vi "Torque_and_Power_and_Doppler.vi"() -> ()   [LabVIEW 2020]
doc: "I. Description:\nThis example demonstrates how to continuously acquire data (Waveform) using the DAQ device's internal clock and an analog slope start trigger.\n\nII. Instructions for Running:\n1. Select the physical channel to correspond to where your signal is input on the DAQ device.\n2. Enter the minimum and maximum voltage ranges.\nNote: For better accuracy try to match the Input Ranges to the expected voltage level of the measured signal.\n3. Set the rate of the acquisition. Also set the Samples to Read control. This will determine how many samples are read each time the while loop iterates. This also determines how many points are plotted on the graph each iteration.\nNote: The rate should be at least twice as fast as the maximum frequency component of the signal being acquired.\n4. Set the source of the Analog Slope Start Trigger.\n5. Set the slope and level of desired analog edge condition.\n\nIII. Block Diagram Steps:\n1. Create an analog input voltage channel.\n2. Set the rate for the sample clock. Additionally, define the sample mode to be continuous.\n3. Define the parameters for an Analog Slope Start Trigger.\n4. Call the Start VI to start the acquisition.\n5. Read the waveform data in a loop until the user hits the stop button or an error occurs.\n6. Call the Clear Task VI to clear the Task.\n7. Use the popup dialog box to display an error if any.\n\nIV. I/O Connections Overview:\nMake sure your signal input terminal matches the Physical Channel I/O control. Also, make sure your analog trigger terminal matches the Trigger Source Control. For further connection information, refer to your hardware reference manual."
uses:
  <extravilib>/ChannelInstances/Tag-bool/Read With Abort.vi
  <extravilib>/ChannelInstances/Tag-bool/Write With Abort.vi
  <extravilib>/ChannelInstances/Tag-bool/Instantiate.vi
  <extravilib>/ChannelInstances/Tag-bool/EndpointRead.vi
  <extravilib>/ChannelInstances/Tag-bool/Endpoint.vi
  <extravilib>/ChannelInstances/Tag-bool.lvlib
panel:
  in  "stop 3":bool
  out "Feet Count":u64
  out "Pulses":u64
  out "Voltage":dynamicdata(graph)
  out "Current":dynamicdata(graph)
  out "Torque":dynamicdata(graph)
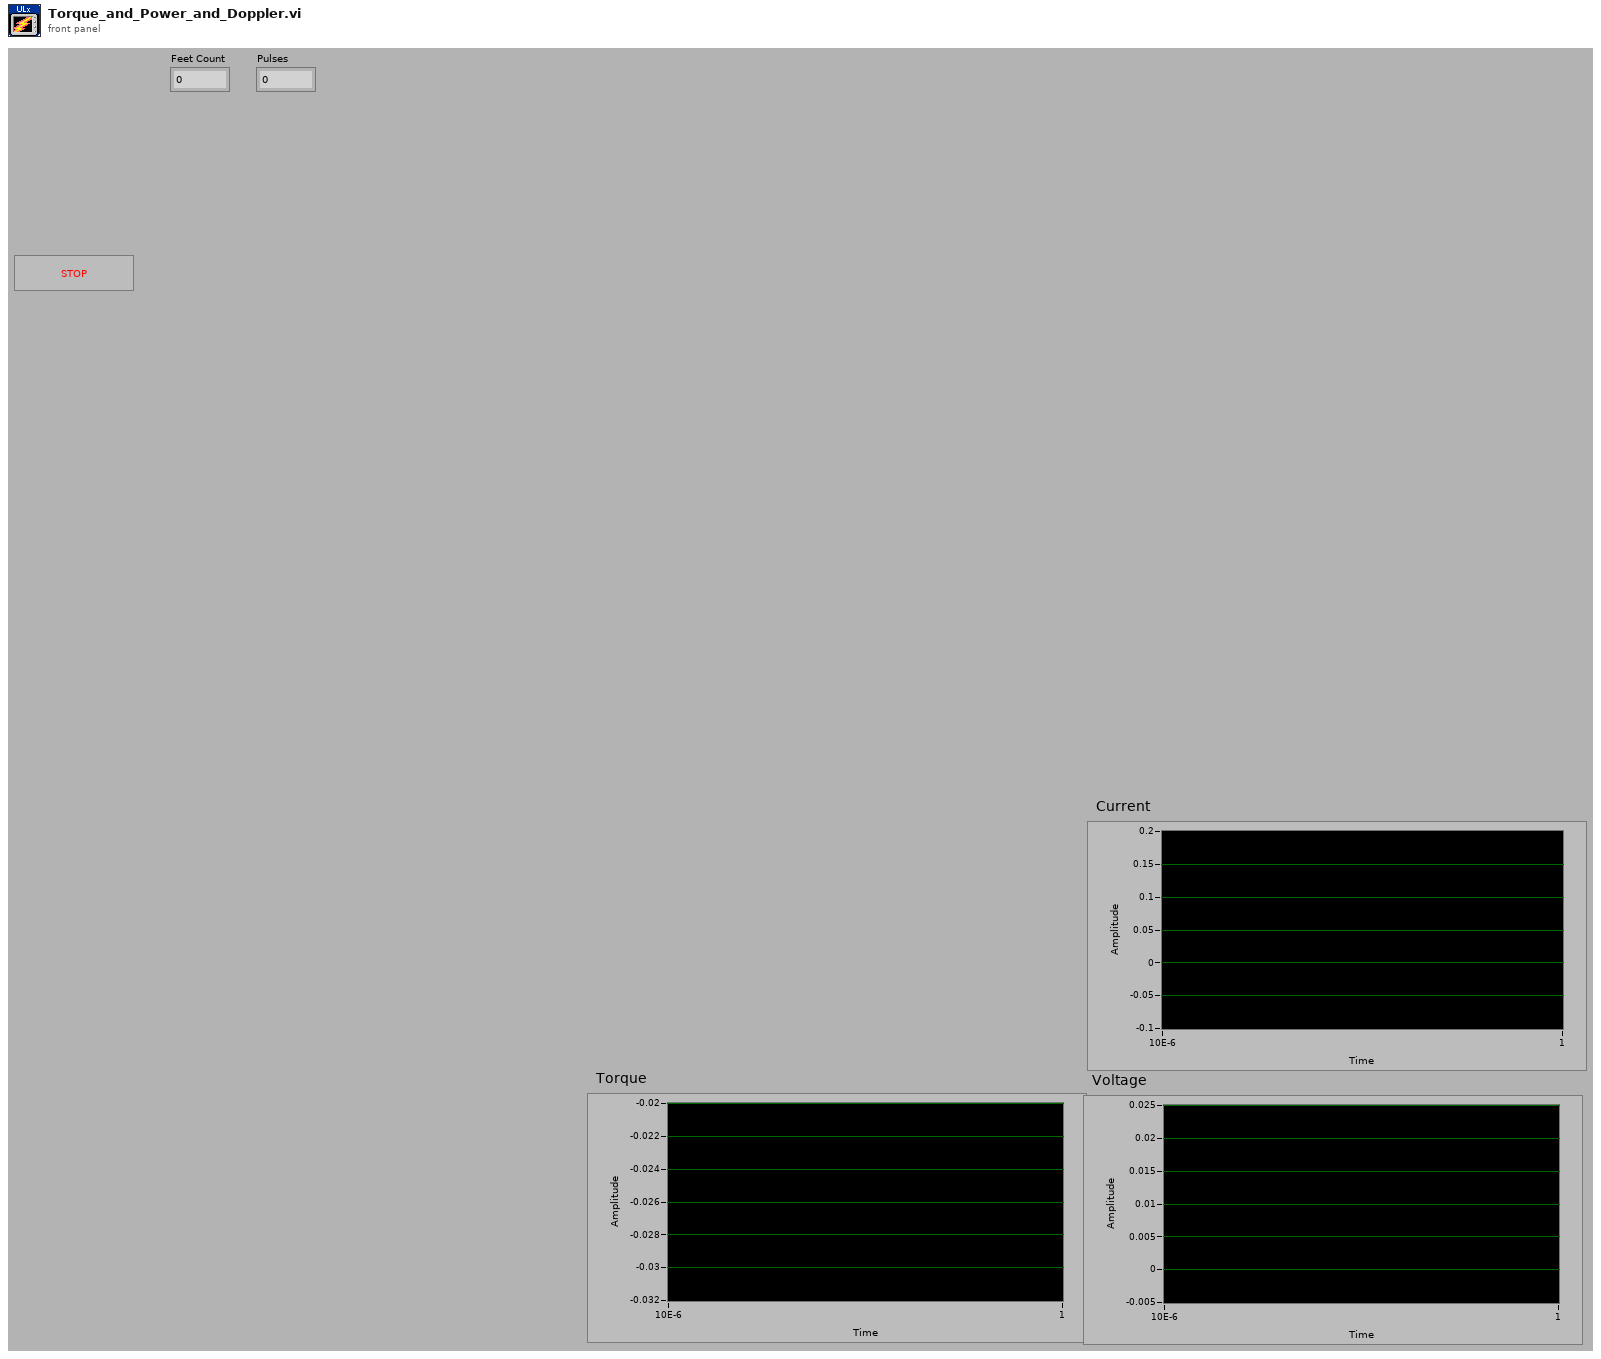
[diagram p1: front panel]
types:
  T1 = typedef "Tag-bool.lvlib/))Channel.ctl" = refnum<queue>
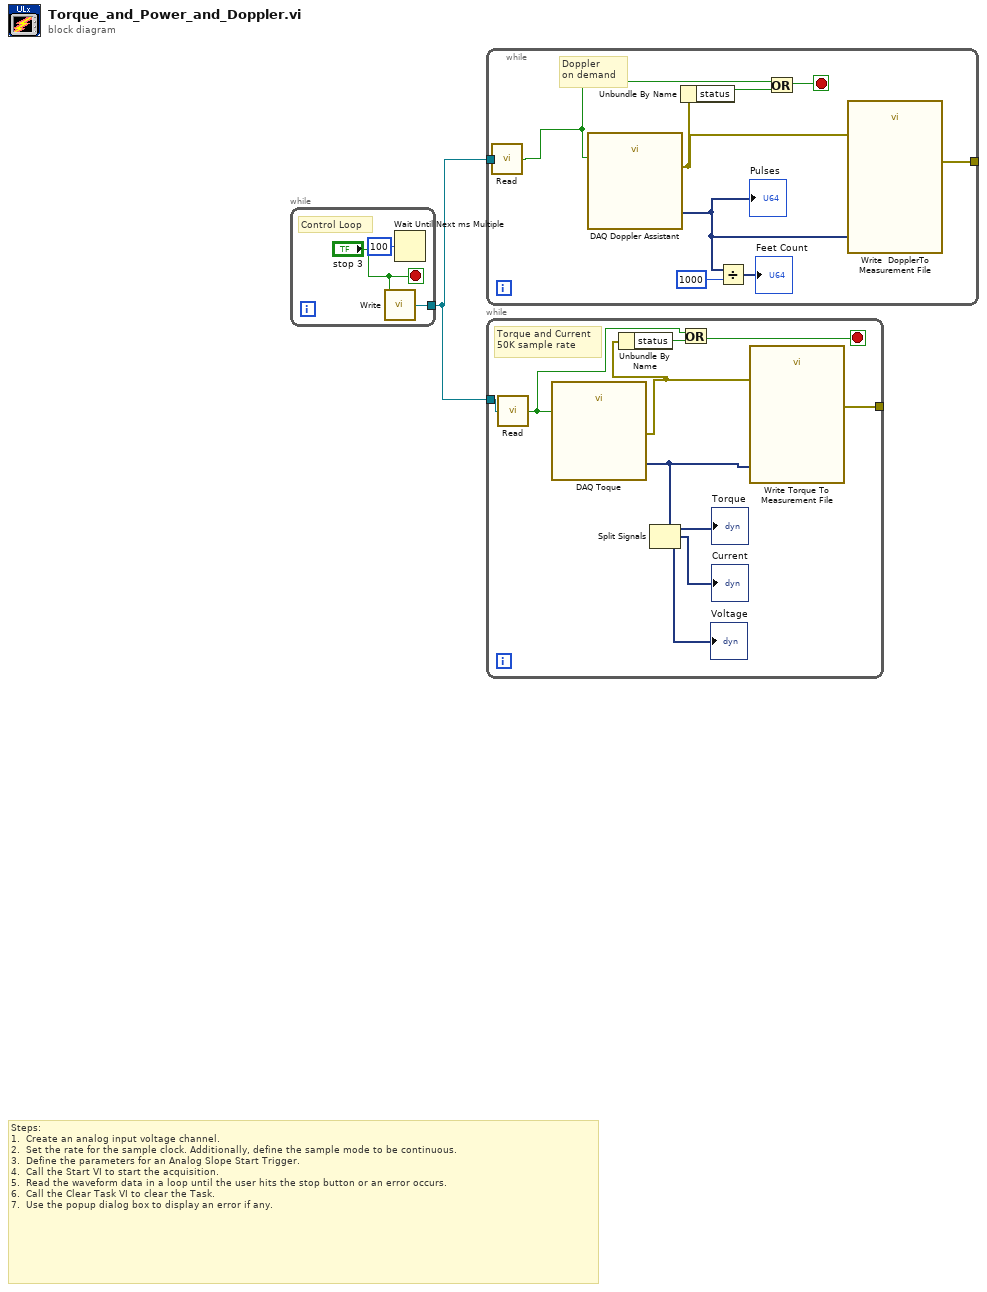
[diagram p0: block diagram]
diagram:
  # "Steps: \n1.  Create an analog input voltage channel.\n2.  Set the rate for the sample clock. Additionally, define the sample mode to be continuous.\n3.  Define the parameters for an Analog Slope Start Trigger.\n4.  Call the Start VI to start the acquisition.\n5.  Read the waveform data in a loop until the user hits the stop button or an error occurs.\n6.  Call the Clear Task VI to clear the Task.\n7.  Use the popup dialog box to display an error if any."
  n1 = while {
    tunnel: [w2] -> w1
    stop <- "stop 3" stop-if-true
    # "Control Loop"
    n2 = call <extravilib>:"Write.vi"("element"="stop 3") -> ("channel"=w2:T1)  [unwired: 1 out]
    n3 = Wait Until Next ms Multiple(millisecond multiple=u32 100 ("millisecond timer value")) -> ()  [unwired: 1 out]
  }
  n4 = while {
    tunnel: [w8] -> _
    tunnel: w1 -> [w5]
    stop <- w13 stop-if-true
    # "Doppler\non demand"
    n5 = call <extravilib>:"Read.vi"("channel"=w5) -> ("element"=w6:bool)  [unwired: 1 in, 1 out]
    n6 = call "DAQ Doppler Assistant"("stop (F)"=w6) -> ("data"=w7:dynamicdata, "error out"=w9:errorcluster)  [unwired: 15 in, 2 out]
    "Pulses" <- w7
    n7 = Unbundle By Name(w9) -> ("status"=w12:bool)
    n8 = Divide(x=w7, y=u64 1000) -> (x/y=→"Feet Count":dynamicdata)
    n9 = Or(x=w6, y=w12) -> (x .or. y?=w13:bool)
    n10 = call "Write  DopplerTo Measurement File"("Signals"=w7, "error in (no error)"=w9) -> ("error out"=w8:errorcluster)  [unwired: 15 in, 2 out]
  }
  n11 = while {
    tunnel: [w20] -> _
    tunnel: w1 -> [w14]
    stop <- w22 stop-if-true
    # "Torque and Current\n50K sample rate"
    n12 = call <extravilib>:"Read.vi"("channel"=w14) -> ("element"=w15:bool)  [unwired: 1 in, 1 out]
    n13 = call "DAQ Toque"("stop (F)"=w15) -> ("data"=w19:dynamicdata, "error out"=w21:errorcluster)  [unwired: 15 in, 2 out]
    n14 = Unbundle By Name(w21) -> ("status"=w23:bool)
    n15 = Split Signals(w19) -> (→"Torque":dynamicdata, →"Current":dynamicdata, →"Voltage":dynamicdata)  [unwired: 3 in]
    n16 = Or(x=w15, y=w23) -> (x .or. y?=w22:bool)
    n17 = call "Write Torque To Measurement File"("Signals"=w19, "error in (no error)"=w21) -> ("error out"=w20:errorcluster)  [unwired: 15 in, 2 out]
  }
